vi "Get Next Event.vi"(5 "Exit Event":string, 7 "event queue in":string[](array[string])) -> (0 "Condition (Exit:F)":bool, 2 "next event":string, 3 "event queue out":string[](array[string]))   [LabVIEW 2018]
doc: "Example of implementing an architecture for interactive LabVIEW applications. See the \"Interactive Architectures Revisited\" article in the LabVIEW Technical Resource newsletter, Spring 1996 issue for more details.\n\nSubscribe to the LabVIEW Technical Resource newsletter!\nContact:\nLTR Publishing\n5614 Anita\nDallas, TX 75206\n(214) 827-9931\nFAX (214) 827-9932\nemail ltrsub@aol.com"
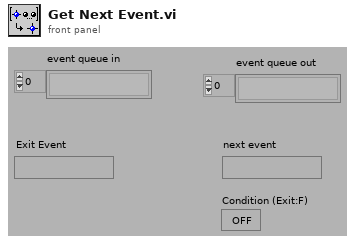
[diagram p1: front panel]
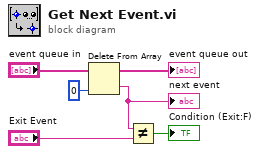
[diagram p0: block diagram]
diagram:
  n1 = Delete From Array(array="event queue in", index=0 ("Index")) -> (deleted portion=w1:string, array with subset deleted=→"event queue out":string[])  [unwired: 1 in]
  "next event" <- w1
  n2 = Not Equal?(x=w1, y="Exit Event") -> (x != y?=→"Condition (Exit:F)":bool)
